vi "gpanel_handle_error.vi"(8 "error in (no error)":errorcluster, 11 "galvo_panel in":refnum<class "galvo_panel.lvclass">) -> (0 "error out":errorcluster, 3 "galvo_panel out":refnum<class "galvo_panel.lvclass">)   [LabVIEW 2015, in "galvo_panel.lvclass"]
uses:
  galvo_panel.lvclass
  galvo_panel.lvclass/galvo_panel.ctl
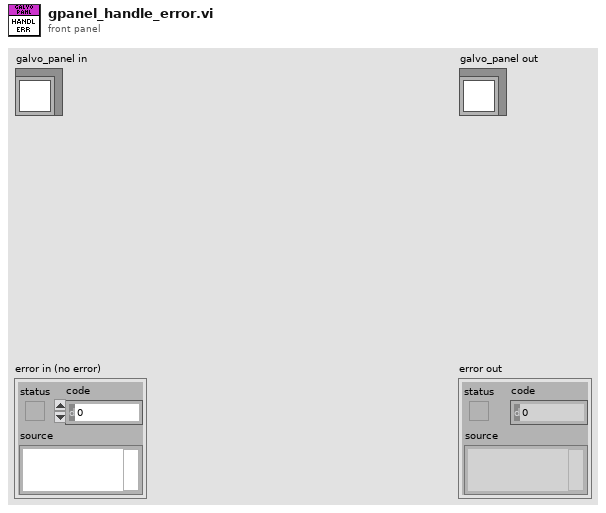
[diagram p1: front panel]
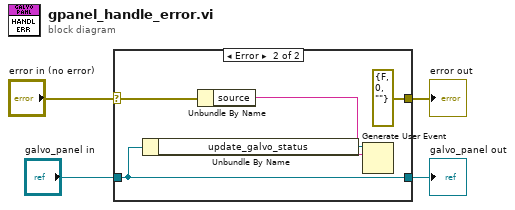
[diagram p0: block diagram]
diagram:
  n1 = case shown="Error" "error in (no error)" {
    selector: "error in (no error)" -> [w5 w9]
    tunnel: [w5 errorcluster {"status"=FALSE, "code"=0, "source"=""} ("error IO")] -> w3
    tunnel: [w6 w11] -> w1
    tunnel: "galvo_panel in" -> [w6 w11]
    frame No Error {
    }
    frame Error {
      n2 = Unbundle By Name(w11) -> ("update_galvo_status"=w10:refnum<user-event>)
      n3 = Unbundle By Name(w9) -> ("source"=w8:string)
      n4 = Generate User Event(user event=w10, event data cluster=w8) -> ()  [unwired: 2 in, 2 out]
    }
  }
  "error out" <- w3
  "galvo_panel out" <- w1
